vi "DCCM Configure Range and Terminal Settings.vi"(0 "DAQmx Task In":refnum<k21>, 5 "Range and Terminal Settings":T1={"Global Settings"={"Min Range (A)"=-10.0, "Max Range (A)"=10.0, "Terminal Configuration"=10083, "Shunt Resistor (Ohm)"=0.001}, "Specific Channel Settings"=[]} {"Specific Channel Settings"."Shunt Resistor (ohms)" format="%#.2p"; "Specific Channel Settings"."Terminal Configuration" items=["RSE"=10083, "NRSE"=10078, "Differential"=10106]; "Specific Channel Settings"."Max Range" format="%#.2p"; "Specific Channel Settings"."Min Range" format="%#.2p"; "Global Settings"."Terminal Configuration" items=["RSE"=10083, "NRSE"=10078, "Differential"=10106]}, 11 "error in (no error)":errorcluster) -> (4 "DAQmx Task Out":refnum<k21>, 15 "error out":errorcluster)   [LabVIEW 2021, in "DAQ_DC-RMS Current Measurement.lvlib"]
doc: "<B>Configure Range and Terminal Settings </B>\n<B>Global Settings </B>configures the range and terminal settings for all analog input voltage channels except the channels specified in the specific channel settings\n\n<B>Specific Channel Settings</B> the range and terminal settings for the physical analog input voltage channels. If the channels are specified in the list, the global settings will be applied."
uses:
  DAQ_DC-RMS Current Measurement.lvlib
  <resource>/objmgr/daqmx.rc
  Typedefs/Specific Channel Settings.ctl
  Typedefs/Range and Terminal Settings.ctl
panel:
  # "Min. Range(A)"
  # "Max. Range(A)"
  # "Terminal Configuration"
  # "Shunt\nResistor(Ohm)"
  # "Physical Channel Name"
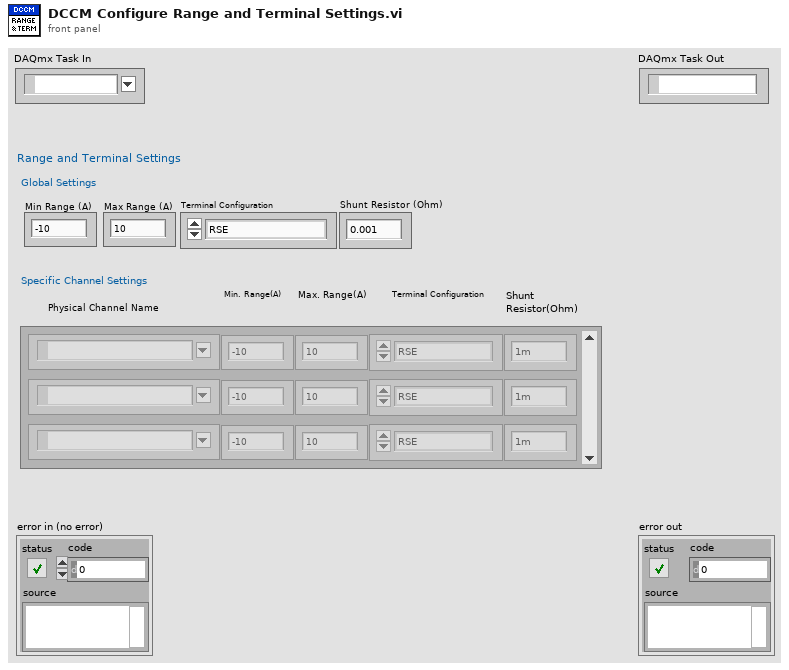
[diagram p1: front panel]
types:
  T1 = typedef "DAQ_DC-RMS Current Measurement.lvlib/Range and Terminal Settings.ctl" = cluster{"Global Settings":cluster{"Min Range (A)":dbl, "Max Range (A)":dbl, "Terminal Configuration":i32, "Shunt Resistor (Ohm)":dbl}, "Specific Channel Settings":T2[]}
  T2 = typedef "DAQ_DC-RMS Current Measurement.lvlib/Specific Channel Settings.ctl" = cluster{"Active Channels":tag, "Min Range":dbl, "Max Range":dbl, "Terminal Configuration":i32, "Shunt Resistor (ohms)":dbl}
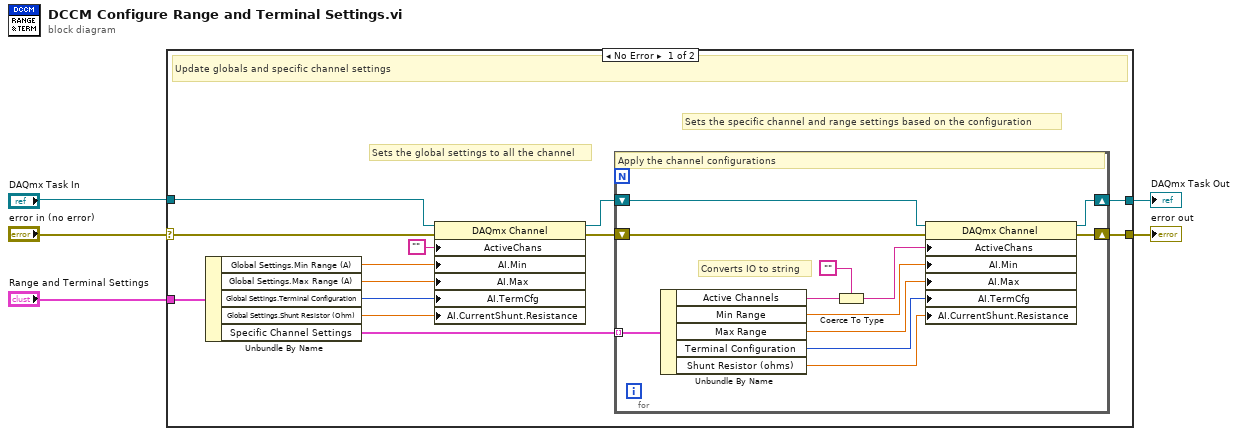
[diagram p0: block diagram]
diagram:
  n1 = case shown="No Error" "error in (no error)" {
    selector: "error in (no error)" -> [w12 w32]
    tunnel: "DAQmx Task In" -> [w14 w31]
    tunnel: "Range and Terminal Settings" -> [w11 _]
    tunnel: [w10 w31] -> w3
    tunnel: [w9 w32] -> w2
    frame No Error {
      # "Sets the specific channel and range settings based on the configuration"
      # "Sets the global settings to all the channel"
      # "Update globals and specific channel settings"
      n2 = Unbundle By Name(w11) -> ("Global Settings.Min Range (A)"=w7:dbl, "Global Settings.Max Range (A)"=w17:dbl, "Global Settings.Terminal Configuration"=w18:i32, "Global Settings.Shunt Resistor (Ohm)"=w6:dbl, "Specific Channel Settings"=w8:T2[])
      n3 = property class="DAQmx Channel"(reference=w14, error in=w12, "ActiveChans"="", "AI.Min"=w7, "AI.Max"=w17, "AI.TermCfg"=w18, "AI.CurrentShunt.Resistance"=w6) -> (reference out=w15:refnum<k21>, error out=w13:errorcluster)
      n4 = for {
        shift-right: [w28] -> w10
        shift-left: w15 -> [w29]
        shift-right: [w30] -> w9
        shift-left: w13 -> [w23]
        tunnel: w8 -> [w26] mode=indexing
        # "Converts IO to string"
        # "Apply the channel configurations"
        n5 = Unbundle By Name(w26) -> ("Active Channels"=w21:tag, "Min Range"=w25:dbl, "Max Range"=w24:dbl, "Terminal Configuration"=w27:i32, "Shunt Resistor (ohms)"=w19:dbl)
        n6 = Coerce To Type(0:w21, 1:"") -> (2:w20:string)
        n7 = property class="DAQmx Channel"(reference=w29, error in=w23, "ActiveChans"=w20, "AI.Min"=w25, "AI.Max"=w24, "AI.TermCfg"=w27, "AI.CurrentShunt.Resistance"=w19) -> (reference out=w28:refnum<k21>, error out=w30:errorcluster)
      }
    }
    frame Error {
      # "Skip settings"
    }
  }
  "DAQmx Task Out" <- w3
  "error out" <- w2
